vi "SetAttributeViString.vi"(7 "AttributeValue":string, 8 "error in (no error)":errorcluster {"code" format="%.0x"}, 9 "AttributeID":u32(ring)=1150090 items=["ACP_DISPLAY_TEXT"=1150090, "CHANNELPOWER_DISPLAY_TITLE"=1190233, "DIGITAL_DEMOD_DISPLAY_TEXT"=1191586, "DIGITAL_DEMOD_SYNC_PATTERN"=1191655, "DIGITAL_DEMOD_TRACE_LIMIT_COMMENT"=1191671, "DIGITAL_DEMOD_TRACE_LIMIT_DESCRIPTION"=1191670, "MONITOR_DISPLAY_TITLE"=1190351, "OCCUPIED_BANDWIDTH_DISPLAY_TEXT"=1190390, "POWER_STATISTICS_DISPLAY_TEXT"=1190433, "SEMASK_DISPLAY_TEXT"=1190491, "SPURIOUS_EMISSIONS_DISPLAY_TEXT"=1190519, "WAVEFORM_DISPLAY_TITLE"=1190543], 10 "RepCapIdentifier":string, 11 "instrument handle":refnum<k15>) -> (0 "error out":errorcluster {"code" format="%.0x"}, 3 "instrument handle out":refnum<k15>)   [LabVIEW 2021, in "Keysight XSAnVMA.lvlib"]
doc: "Sets a String attribute from the instrument driver.\nThe following Attributes are supported:\n\nACP_DISPLAY_TEXT\nCHANNELPOWER_DISPLAY_TITLE\nDIGITAL_DEMOD_DISPLAY_TEXT\nDIGITAL_DEMOD_SYNC_PATTERN\nDIGITAL_DEMOD_TRACE_LIMIT_COMMENT\nDIGITAL_DEMOD_TRACE_LIMIT_DESCRIPTION\nMONITOR_DISPLAY_TITLE\nOCCUPIED_BANDWIDTH_DISPLAY_TEXT\nPOWER_STATISTICS_DISPLAY_TEXT\nSEMASK_DISPLAY_TEXT\nSPURIOUS_EMISSIONS_DISPLAY_TEXT\nWAVEFORM_DISPLAY_TITLE"
uses:
  <instrlib>/Keysight XSAnVMA/Keysight XSAnVMA.lvlib
  KtXSAnVMA_64.dll
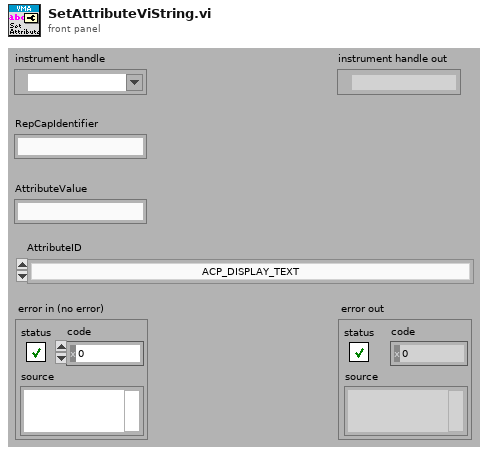
[diagram p1: front panel]
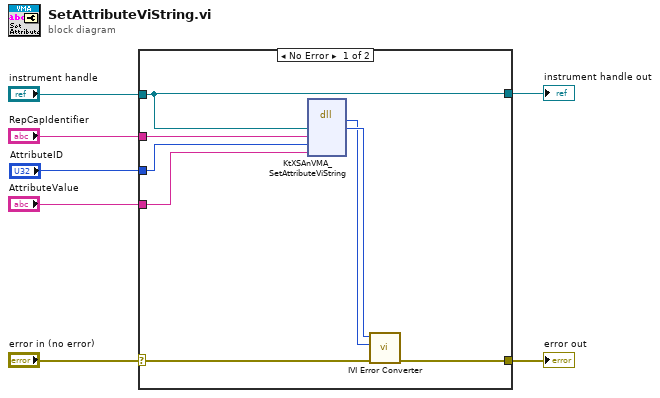
[diagram p0: block diagram]
diagram:
  n1 = case shown="No Error" "error in (no error)" {
    selector: "error in (no error)" -> [w13 w17]
    tunnel: [w12 w17] -> w7
    tunnel: "instrument handle" -> [w8 w16]
    tunnel: "RepCapIdentifier" -> [w11 _]
    tunnel: "AttributeID" -> [w10 _]
    tunnel: "AttributeValue" -> [w9 _]
    tunnel: [w8 w16] -> w2
    frame No Error {
      n2 = dll-call lib="KtXSAnVMA**.dll" fn="KtXSAnVMA_SetAttributeViString"("Vi"=w8, "RepCapIdentifier"=w11, "AttributeID"=w10, "AttributeValue"=w9) -> ("return type"=w14:i32, "Vi"=w15:u32)  [unwired: 6 in, 2 out]
      n3 = call <instrlib>:"IVI Error Converter.vi"("error in (no error)"=w13, "IVI error code (0)"=w14, "instrument handle"=w15) -> ("error out"=w12:errorcluster)  [unwired: 7 in, 1 out]
    }
    frame Error {
    }
  }
  "error out" <- w7
  "instrument handle out" <- w2
